vi "Read Sim Axis Data.vi"(8 "error in (no error)":errorcluster, 11 "Parent SIM Motion Controller in":refnum<class "FINE SIM Motion Axis.lvclass">) -> (0 "error out":errorcluster, 2 "Sim Axis Data":T1={"Axis Parameters"={"Moving"=FALSE, "Homed"=FALSE, "Desired Position"=0.0, "Current Positon"=0.0, "Current Speed"=0.0, "Home Status"=enum."Inital Home Motion"}, "Time Stamp"=timestamp(0 s since 1904-01-01), "Settings"={"Axis Name"="", "Axis Settings"={"Speed"=0.0, "Acceleration"=0.0}}}, 3 "Parent SIM Motion Controller out":refnum<class "FINE SIM Motion Axis.lvclass">)   [LabVIEW 2022 SP3, in "FINE SIM Motion Axis.lvclass"]
uses:
  FINE SIM Motion Axis.lvclass
  TypeDefs/Axis Data.ctl
  TypeDefs/Axis Parameters.ctl
  TypeDefs/Homing Status.ctl
  TypeDefs/Axis Settings.ctl
  FINE SIM Motion Axis.lvclass/FINE SIM Motion Axis.ctl
  TypeDefs/Settings.ctl
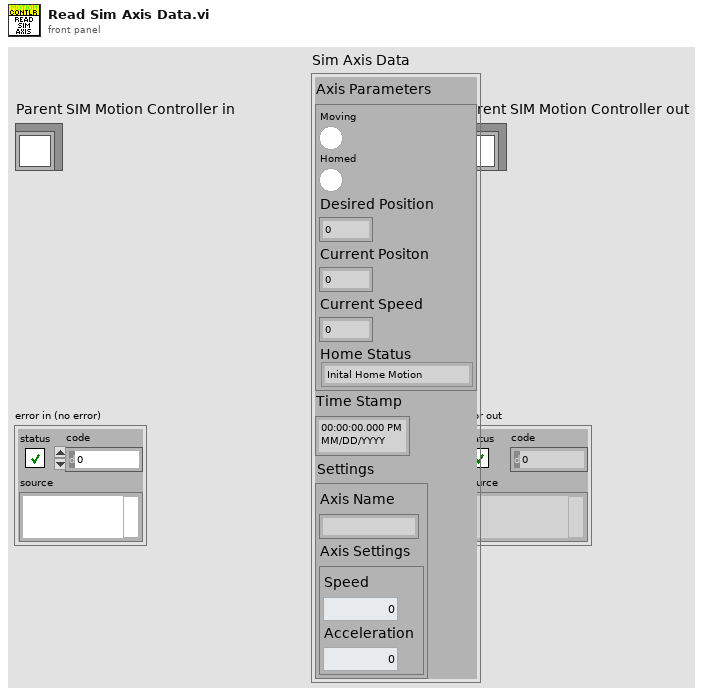
[diagram p1: front panel]
types:
  T1 = typedef "FINE SIM Motion Axis.lvclass/Axis Data.ctl" = cluster{"Axis Parameters":T2, "Time Stamp":timestamp, "Settings":T4}
  T2 = typedef "FINE SIM Motion Axis.lvclass/Axis Parameters.ctl" = cluster{"Moving":bool, "Homed":bool, "Desired Position":dbl, "Current Positon":dbl, "Current Speed":dbl, "Home Status":T3}
  T3 = typedef "FINE SIM Motion Axis.lvclass/Homing Status.ctl" = enum16{"Idle", "Inital Home Motion", "Final Home Motion", "Done Homing"}
  T4 = typedef "FINE SIM Motion Axis.lvclass/Settings.ctl" = cluster{"Axis Name":string, "Axis Settings":T5}
  T5 = typedef "FINE SIM Motion Axis.lvclass/Axis Settings.ctl" = cluster{"Speed":dbl, "Acceleration":dbl}
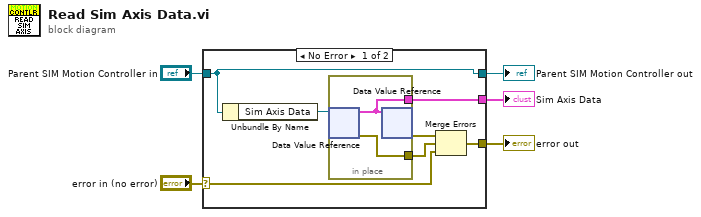
[diagram p0: block diagram]
diagram:
  n1 = case shown="No Error" "error in (no error)" {
    selector: "error in (no error)" -> [w8 w15]
    tunnel: [w7 w15] -> w4
    tunnel: [w12 w16] -> w2
    tunnel: "Parent SIM Motion Controller in" -> [w12 w16]
    tunnel: [w6 _] -> w1
    frame No Error {
      n2 = Unbundle By Name(w12) -> ("Sim Axis Data"=w11:refnum<data-value>)
      n3 = in-place {
        in-place-border: [w14] -> w9
        in-place-border: [w13] -> w6
        n4 = in-place-dvr #1(w11) -> (w13:T1, w14:errorcluster)
        n5 = in-place-dvr #1(w13) -> (w10:errorcluster)  [unwired: 1 out]
      }
      n6 = Merge Errors(w10, w9, w8) -> (w7:errorcluster)
    }
    frame Error {
    }
  }
  "error out" <- w4
  "Parent SIM Motion Controller out" <- w2
  "Sim Axis Data" <- w1
